vi "Autonomous Independent.vi"() -> ()   [LabVIEW 2017]
doc: "This VI is called when autonomous begins, and will automatically be terminated when autonomous ends. You can carry out timed or sensor driven robot movement independently without needing to return to the caller."
uses:
  <vilib>/Rock Robotics/WPI/Utilities/WPI_GetSetVariantRefNum.vi
  <vilib>/Rock Robotics/Network Tables/NT Read String.vi
  <vilib>/Rock Robotics/Network Tables/NT Write Numeric Array.vi
  <vilib>/Rock Robotics/Network Tables/NT Read Number.vi
  <vilib>/Rock Robotics/Network Tables/NT Read String Array.vi
panel:
  out "x = y?":bool
  out "Switch":string
  out "Scale Compare?":bool
  out "Scale":string
  out "Setpoint2":dbl
  out "Setpoint":dbl
  # "Be sure to right-click and choose Data Operations>>Make Current Value default if you want to save the array values with the VI"
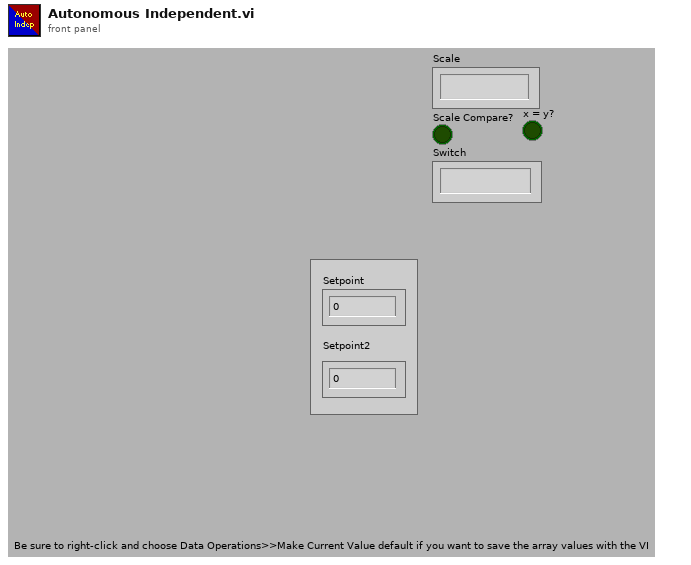
[diagram p1: front panel]
types:
  T1 = typedef "WPI_JoystickDevRef.ctl" = cluster{"Device":T2}
  T2 = typedef "WPI_JoystickDeviceEnum.ctl" = enum16{"USB 0", "USB 1", "USB 2", "USB 3", "USB 4", "USB 5"}
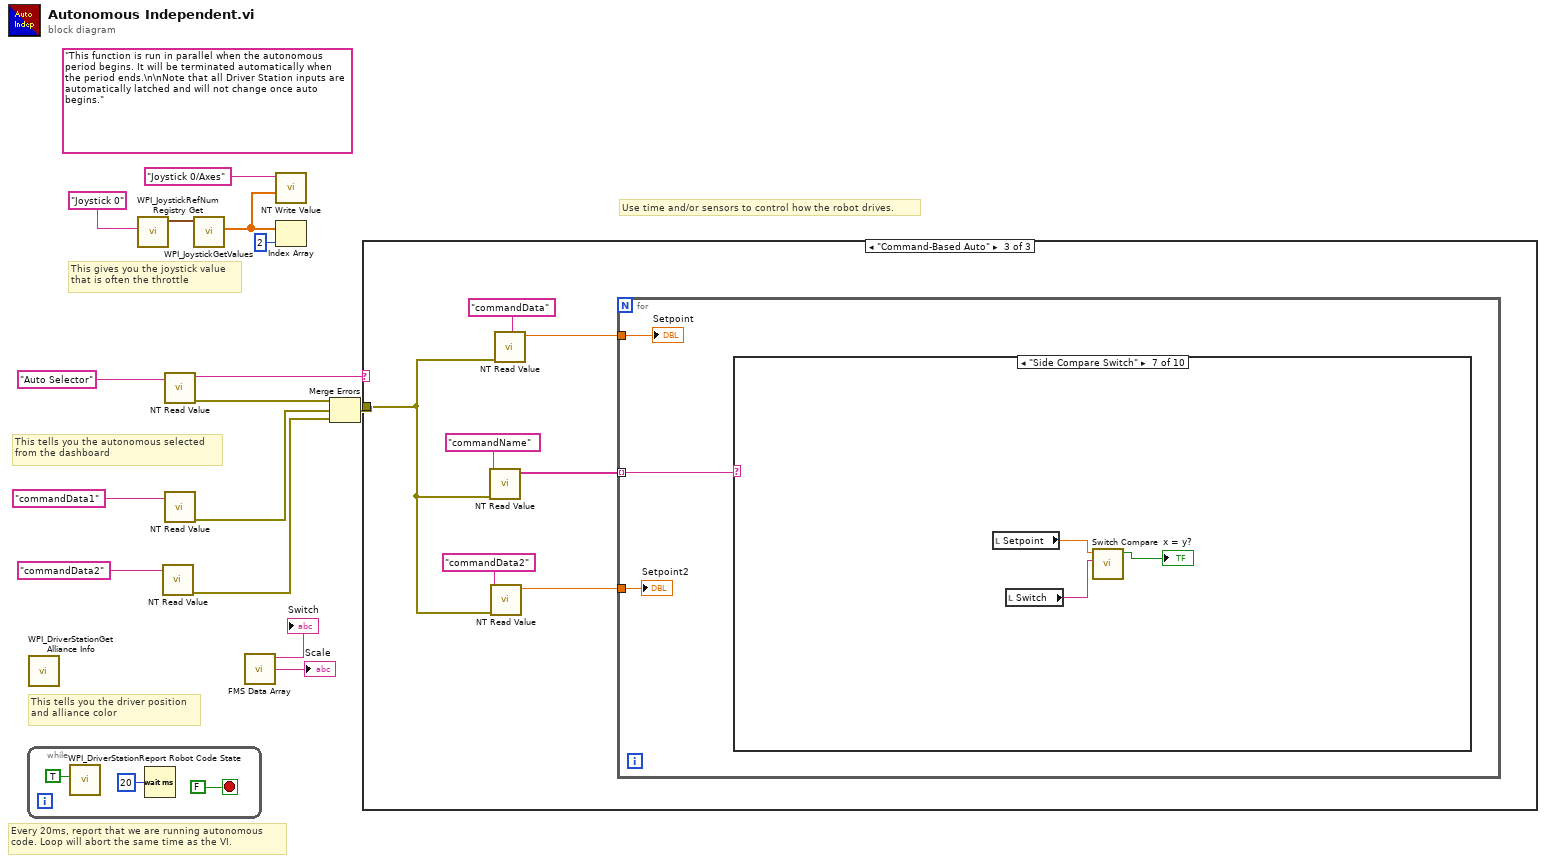
[diagram p0: block diagram]
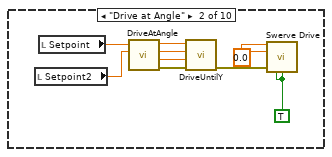
[diagram p5: hidden frame]
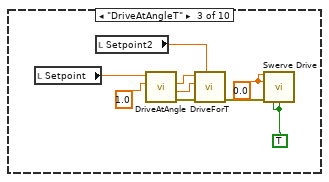
[diagram p6: hidden frame]
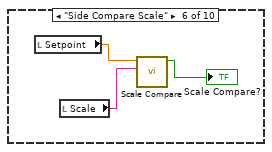
[diagram p9: hidden frame]
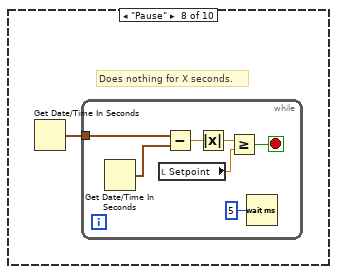
[diagram p10: hidden frame]
diagram:
  (unwired) "This function is run in parallel when the autonomous period begins. It will be terminated automatically when the period ends.\n\nNote that all Driver Station inputs are automatically latched and will not change once auto begins."
  # "This tells you the autonomous selected\nfrom the dashboard"
  # "Every 20ms, report that we are running autonomous\ncode. Loop will abort the same time as the VI."
  # "This gives you the joystick value\nthat is often the throttle"
  # "Use time and/or sensors to control how the robot drives."
  # "This tells you the driver position\nand alliance color"
  n1 = while {
    stop <- FALSE stop-if-true
    n2 = call <vilib>:"WPI_DriverStationReport Robot Code State.vi"("Autonomous"=TRUE) -> ()  [unwired: 10 in, 1 out]
    n3 = Wait (ms)(milliseconds to wait=u32 20) -> ()  [unwired: 1 out]
  }
  n4 = call <vilib>:"WPI_DriverStationGet Alliance Info.vi"() -> ()  [unwired: 12 out]
  n5 = call <vilib>:"WPI_JoystickRefNum Registry Get.vi"("refnum name"="Joystick 0") -> ("JoystickDevRef"=w14:T1)  [unwired: 1 in, 9 out]
  n6 = call-poly <vilib>:"NT Read Value.vi"("Name"="commandData2") -> ("error out"=w3:errorcluster)  [unwired: 9 in, 1 out]
  n7 = call-poly <vilib>:"NT Read Value.vi"("Name"="Auto Selector") -> ("error out"=w8:errorcluster, "String"=w9:string)  [unwired: 9 in]
  n8 = call-poly <vilib>:"NT Read Value.vi"("Name"="commandData1") -> ("error out"=w7:errorcluster)  [unwired: 9 in, 1 out]
  n9 = call <vilib>:"WPI_JoystickGetValues.vi"("JoystickDevRef"=w14) -> ("Axes"=w11:dbl[])  [unwired: 6 in, 4 out]
  n10 = call "FMS Data Array.vi"() -> ("Scale"=→"Scale":string, "Switch"=→"Switch":string)  [unwired: 9 in, 1 out]
  n11 = call-poly <vilib>:"NT Write Value.vi"("Numeric Array"=w11, "Name"="Joystick 0/Axes") -> ()  [unwired: 9 in, 1 out]
  n12 = Index Array(array=w11, index=2) -> ()  [unwired: 1 out]
  n13 = Merge Errors(w8, w7, w3) -> (w5:errorcluster)
  n14 = case shown="\"Command-Based Auto\"" w9 {
    tunnel: w5 -> [_ _ w20]
    frame Default {
      # "You can put your main auto here, or you can right-click on the case and make any\nother frame be the default case."
      # "This is the frame that will execute if no selection is made, or if it is not recognized"
    }
    frame "Swerve Calibration" {
    }
    frame "Command-Based Auto" {
      n15 = call-poly <vilib>:"NT Read Value.vi"("error in"=w20, "Name"="commandName") -> ("String Array"=w22:string[])  [unwired: 8 in, 1 out]
      n16 = call-poly <vilib>:"NT Read Value.vi"("error in"=w20, "Name"="commandData2") -> ("Numeric"=w19:dbl)  [unwired: 8 in, 1 out]
      n17 = call-poly <vilib>:"NT Read Value.vi"("error in"=w20, "Name"="commandData") -> ("Numeric"=w23:dbl)  [unwired: 8 in, 1 out]
      n18 = for {
        tunnel: w23 -> [w28]
        tunnel: w22 -> [w27] mode=indexing
        tunnel: w19 -> [w26]
        n19 = case shown="\"Side Compare Switch\"" w27 {
          frame "Turn to Angle" {
          }
          frame "Drive at Angle" {
            w29 = TRUE ("Autonomous?")
            w30 = 0.0 ("X")
            n20 = local read "Setpoint2"() -> (w36:dbl)
            n21 = local read "Setpoint"() -> (w37:dbl)
            n22 = call "DriveAtAngle.vi"("Target Angle"=w37, "Distance"=w36) -> ("y-axis distance"=w32:dbl, "x"=w33:dbl, "y"=w34:dbl, "Error Out"=w35:errorcluster)  [unwired: 5 in]
            n23 = call "DriveUntilY.vi"("error in"=w35, "y"=w34, "x"=w33, "y-axis distance"=w32) -> ("error out"=w31:errorcluster)  [unwired: 7 in]
            n24 = call "Swerve Drive.vi"("X"=w30, "Y"=w30, "Error In"=w31, "Robot Centric?"=w29, "Autonomous?"=w29) -> ()  [unwired: 6 in, 5 out]
          }
          frame "DriveAtAngleT" {
            w38 = TRUE ("Autonomous?")
            w39 = 0.0 ("X")
            n25 = local read "Setpoint"() -> (w46:dbl)
            n26 = local read "Setpoint2"() -> (w41:dbl)
            n27 = call "DriveAtAngle.vi"("Target Angle"=w46, "Distance"=1.0) -> ("x"=w42:dbl, "y"=w43:dbl, "Error Out"=w44:errorcluster)  [unwired: 5 in, 1 out]
            n28 = call "DriveForT.vi"("time(sec)"=w41, "Error In"=w44, "y"=w43, "x"=w42) -> ("Error Out"=w40:errorcluster)  [unwired: 7 in]
            n29 = call "Swerve Drive.vi"("X"=w39, "Y"=w39, "Error In"=w40, "Robot Centric?"=w38, "Autonomous?"=w38) -> ()  [unwired: 6 in, 5 out]
          }
          frame "Lift Main" {
          }
          frame "Drive Until Distance" {
          }
          frame "Side Compare Scale" {
            n30 = local read "Setpoint"() -> (w48:dbl)
            n31 = local read "Scale"() -> (w49:string)
            n32 = call "Scale Compare.vi"("Scale in"=w49, "Setpoint in"=w48) -> ("Scale Compare?"=→"Scale Compare?":bool)  [unwired: 9 in]
          }
          frame "Side Compare Switch" {
            n33 = local read "Setpoint"() -> (w51:dbl)
            n34 = local read "Switch"() -> (w50:string)
            n35 = call "Switch Compare.vi"("Switch"=w50, "Setpoint"=w51) -> ("Boolean"=→"x = y?":bool)  [unwired: 9 in]
          }
          frame "Pause" {
            # "Does nothing for X seconds."
            n36 = Get Date/Time In Seconds() -> (seconds since 1Jan1904=w53:timestamp)
            n37 = while {
              tunnel: w53 -> [w60]
              stop <- w55 stop-if-true
              n38 = Get Date/Time In Seconds() -> (seconds since 1Jan1904=w59:timestamp)
              n39 = local read "Setpoint"() -> (w56:dbl)
              n40 = Subtract(x=w60, y=w59) -> (x-y=w58:dbl)
              n41 = Absolute Value(x=w58) -> (abs(x)=w57:dbl)
              n42 = Greater Or Equal?(x=w57, y=w56) -> (x >= y?=w55:bool)
              n43 = Wait (ms)(milliseconds to wait=u32 5) -> ()  [unwired: 1 out]
            }
          }
          frame Default {
          }
          frame "Drive to Distance" {
          }
        }
        "Setpoint" <- w28
        "Setpoint2" <- w26
      }
    }
  }
